vi "Setup Y Tovey.vi"(8 "error in (no error)":errorcluster, 10 "Model in":refnum<class "Model.lvclass">, 11 "Boot Loader in":refnum<class "Boot Loader.lvclass">) -> (0 "error out":errorcluster, 2 "Model out":refnum<class "Model.lvclass">, 3 "Boot Loader out":refnum<class "Boot Loader.lvclass">)   [LabVIEW 2016]
uses:
  Common_SerialProtocols/SerialProtocolFactory/SerialProtocolFactory/SerialProtocolFactory.lvclass
  Common_SerialProtocols/SerialCommunicator/SerialCommunicator.lvclass
  TEI-9150/Tovey 9150.lvclass
  Boot Loader.lvclass
  C:/CODE/ts_HPMT/Common_SerialProtocols/SerialProtocolFactory/ISerialProtocolFactory/ISerialProtocolFactory.lvclass
  Model/Model.lvclass
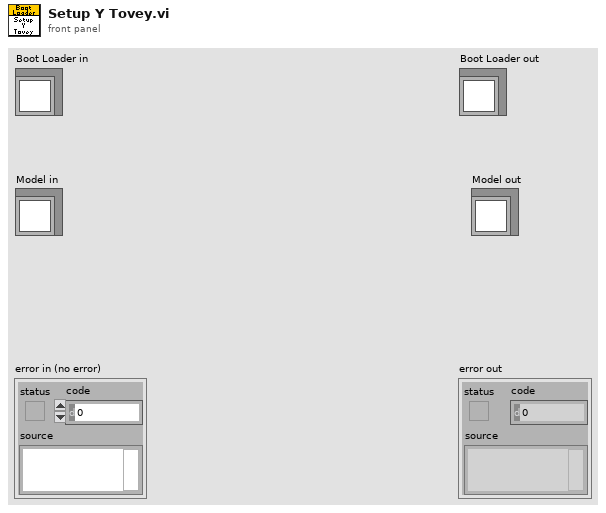
[diagram p1: front panel]
types:
  T1 = typedef "SerialProtocols.lvlib/SerialConfig.ctl" = cluster{"Serial Protocol":T2, "Protocol Parameters":T3, "Serial Message Parameters":T4}
  T2 = typedef "SerialProtocols.lvlib/SerialProtocol.ctl" = enum16{"RS232", "RS485", "SerialSimulator"}
  T3 = typedef "SerialProtocols.lvlib/ProtocolParameters.ctl" = cluster{"VISA resource name":refnum<visa-resource-name>, "Baud Rate":u32, "Data Bits":u16, "Parity":enum16{"None", "Odd", "Even", "Mark", "Space"}, "Flow Control":u16, "Stop Bits":u16, "Timeout (ms)":u32}
  T4 = typedef "SerialProtocols.lvlib/SerialMessageParameters.ctl" = cluster{"Byte Count":u32, "Enable Termination Character":bool, "Termination Char":u8}
  T5 = typedef "HPMT_Typedefs.lvlib/ConnectionSettings.ctl" = cluster{"ILC Port":refnum<visa-resource-name>, "Tovey X Port":refnum<visa-resource-name>, "Tovey Y Port":refnum<visa-resource-name>, "Tovey Z Port":refnum<visa-resource-name>, "Tovey X Protocol":T2, "Tovey Y Protocol":T2, "Tovey Z Protocol":T2, "Tovey X Address":u8, "Tovey Y Address":u8, "Tovey Z Address":u8}
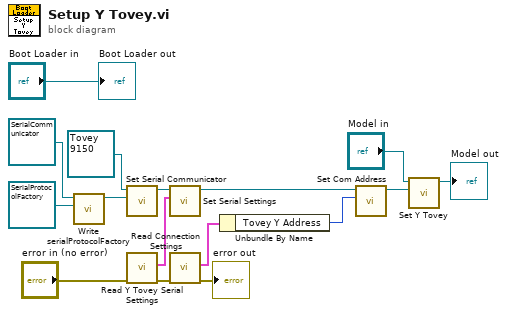
[diagram p0: block diagram]
diagram:
  n1 = call "Write serialProtocolFactory.vi"("serialProtocolFactory"=refnum<class "SerialProtocolFactory.lvclass"> refnum ("SerialCommFactory.lvclass"), "SerialCommunicator in"=refnum<class "SerialCommunicator.lvclass"> refnum ("SerialProtocols.lvlib:SerialCommunicator.lvclass")) -> ("SerialCommunicator out"=w13:refnum<class "SerialCommunicator.lvclass">)  [unwired: 9 in]
  n2 = call "Set Serial Communicator.vi"("SerialProtocols.lvlib:SerialCommunicator.lvclass"=w13, "Tovey9150 in"=refnum<class "Tovey 9150.lvclass"> refnum ("Tovey 9150.lvclass")) -> ("Tovey9150 out"=w11:refnum<class "Tovey 9150.lvclass">)  [unwired: 9 in]
  n3 = call "Read Y Tovey Serial Settings.vi"("error in (no error)"="error in (no error)") -> ("error out"=w7:errorcluster, "Serial"=w4:T1)  [unwired: 8 in, 1 out]
  n4 = call "Set Serial Settings.vi"("Serial Settings"=w4, "Tovey9150 in"=w11) -> ("Tovey9150 out"=w10:refnum<class "Tovey 9150.lvclass">)  [unwired: 9 in]
  n5 = call "Read Connection Settings.vi"("error in (no error)"=w7) -> ("error out"=→"error out":errorcluster, "Connection Settings"=w9:T5)  [unwired: 8 in, 1 out]
  n6 = Unbundle By Name(w9) -> ("Tovey Y Address"=w8:u8)
  n7 = call "Set Com Address.vi"("Com Address"=w8, "Tovey9150 in"=w10) -> ("Tovey9150 out"=w1:refnum<class "Tovey 9150.lvclass">)  [unwired: 9 in]
  n8 = call "Set Y Tovey.vi"("Y Tovey"=w1, "Model in"="Model in") -> ("Model out"=→"Model out":refnum<class "Model.lvclass">)  [unwired: 9 in]
  "Boot Loader out" <- "Boot Loader in"
